vi "USB6343_Control.vi"(11 "monitor buff":refnum<vi>) -> (0 "error out":errorcluster, 3 "msg interface":refnum<user-event>)   [LabVIEW 2013]
uses:
  <vilib>/DAQmx/write.llb/DAQmx Write.vi
  <vilib>/DAQmx/write.llb/DAQmx Write (Digital 1D Bool NChan 1Samp 1Line).vi
  <vilib>/DAQmx/write.llb/DAQmx Write (Analog 1D DBL NChan 1Samp).vi
  <vilib>/DAQmx/read.llb/DAQmx Read.vi
  <vilib>/DAQmx/read.llb/DAQmx Read (Analog 1D DBL NChan 1Samp).vi
  <vilib>/DAQmx/miscellaneous.llb/DAQmx Fill In Error Info.vi
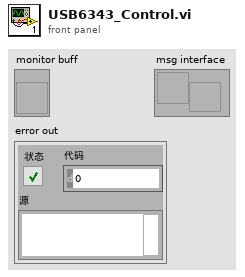
[diagram p1: front panel]
types:
  T1 = cluster{"cmd":string, "value":dbl, "result ":refnum<vi>, "channel":i32, "on/off":bool}
  T2 = cluster{"AI Task":refnum<k21>, "AO Task":refnum<k21>, "DO Task":refnum<k21>}
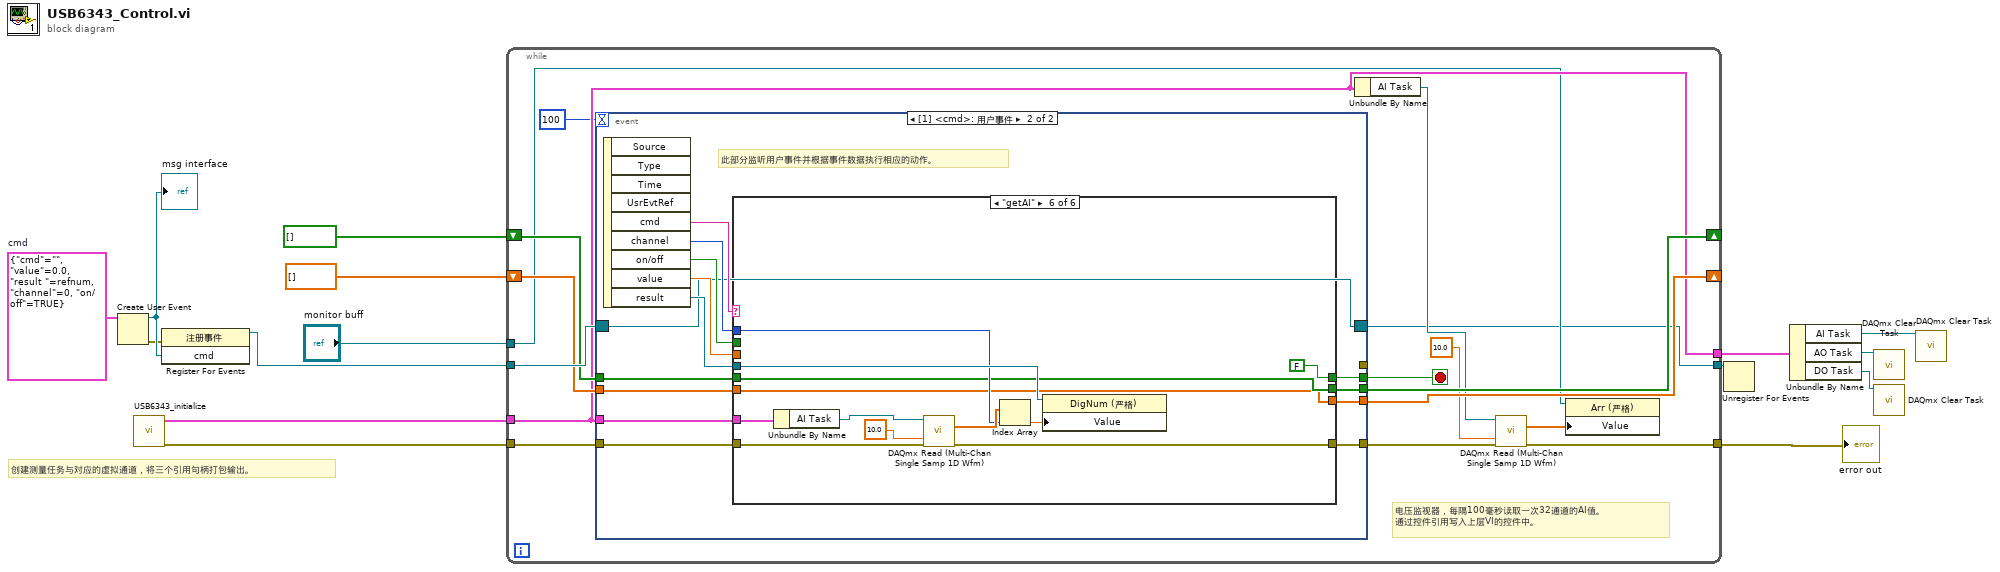
[diagram p0: block diagram]
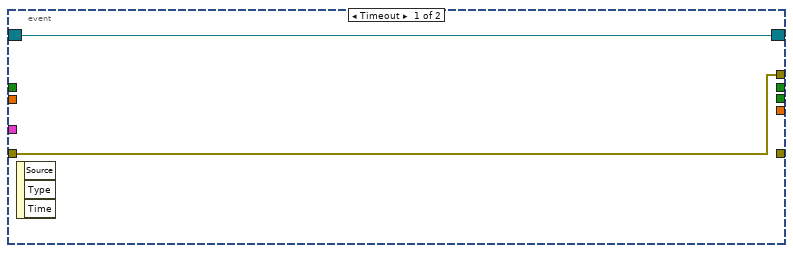
[diagram p2: hidden frame]
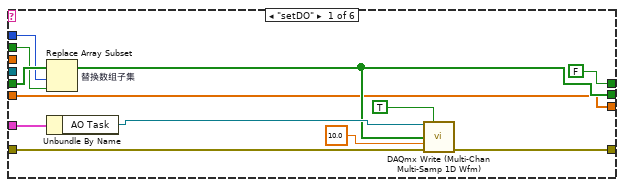
[diagram p3: hidden frame]
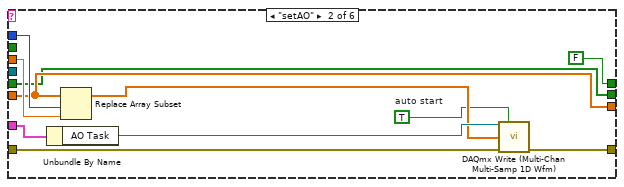
[diagram p4: hidden frame]
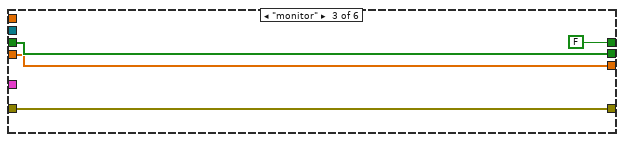
[diagram p5: hidden frame]
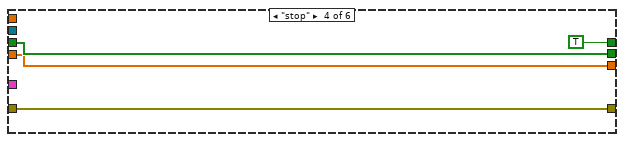
[diagram p6: hidden frame]
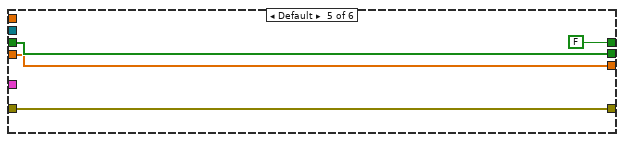
[diagram p7: hidden frame]
diagram:
  w10 = T1 {"cmd"="", "value"=0.0, "result "=refnum, "channel"=0, "on/off"=TRUE}  # cmd
  # "创建测量任务与对应的虚拟通道，将三个引用句柄打包输出。"
  n1 = Create User Event(user event datatype=w10) -> (user event=w15:refnum<user-event>, error out=w14:errorcluster)  [unwired: 1 in]
  "msg interface" <- w15
  n2 = call "USB6343_initialize.vi"() -> ("error out"=w12:errorcluster, "Tasks"=w13:T2)  [unwired: 10 in]
  n3 = register-events(error in=w14, w15) -> (reference out=w11:refnum<event-registration>)  [unwired: 1 in, 1 out]
  n4 = while {
    tunnel: w13 -> [w24]
    tunnel: w12 -> [w31]
    tunnel: w11 -> [w30]
    shift-right: [w28] -> _
    shift-left: bool[] [] ("data") -> [w29]
    tunnel: [w24] -> w8
    shift-right: [w25] -> _
    shift-left: dbl[] [] ("data") -> [w26]
    tunnel: "monitor buff" -> [w20]
    tunnel: [w18] -> w3
    tunnel: [w16] -> w1
    stop <- w27 stop-if-true
    # "电压监视器，每隔100毫秒读取一次32通道的AI值。\n通过控件引用写入上层VI的控件中。"
    n5 = event shown="[1] <cmd>: 用户事件" {
      selector: w30 -> [w32 w34]
      dyn-events: [w32 w34] -> w16
      timeout: 100 -> [_ _]
      tunnel: w24 -> [_ w46]
      tunnel: [w33 _] -> _
      tunnel: w31 -> [w33 w45]
      tunnel: w29 -> [_ w44]
      tunnel: [_ w42] -> w28
      tunnel: [_ w40] -> w27
      tunnel: w26 -> [_ w39]
      tunnel: [_ w37] -> w25
      tunnel: [_ w35] -> w21
      event Timeout {
        n6 = event-data() -> ()  [unwired: 1 in, 3 out]
      }
      event User Event {
        # "此部分监听用户事件并根据事件数据执行相应的动作。"
        n7 = event-data() -> ("cmd"=w41:string, "channel"=w47:i32, "on/off"=w43:bool, "value"=w38:dbl, "result"=w36:refnum<vi>)  [unwired: 1 in, 4 out]
        n8 = case shown="\"getAI\"" w41 {
          tunnel: w47 -> [w53 w68 _ _ _ w88]
          tunnel: w46 -> [w59 w70 _ _ _ w94]
          tunnel: w45 -> [w56 w60 w71 w75 w79 w90]
          tunnel: w44 -> [w54 w65 w74 w78 w82 w86]
          tunnel: w43 -> [w52 _ _ _ _ _]
          tunnel: [w51 w65 w74 w78 w82 w86] -> w42
          tunnel: [FALSE FALSE FALSE TRUE FALSE FALSE] -> w40
          tunnel: w39 -> [w49 w66 w73 w76 w80 w85]
          tunnel: w38 -> [_ w67 _ _ _ _]
          tunnel: [w49 w66 w73 w76 w80 w85] -> w37
          tunnel: w36 -> [_ _ _ _ _ w92]
          tunnel: [w48 w61 w71 w75 w79 w83] -> w35
          frame "setDO" {
            n9 = Replace Array Subset "替换数组子集"(array=w54, new element=w52, index=w53) -> (w51:bool[])
            n10 = Unbundle By Name(w59) -> ("AO Task"=w58:refnum<k21>)
            n11 = call-poly "DAQmx Write (Multi-Chan Multi-Samp 1D Wfm).vi"("task/channels in"=w58, "auto start"=TRUE, "data"=w51, "timeout"=10.0, "error in"=w56) -> ("error out"=w48:errorcluster)  [unwired: 8 in, 2 out]
          }
          frame "setAO" {
            w63 = TRUE  # auto start
            n12 = Unbundle By Name(w70) -> ("AO Task"=w69:refnum<k21>)
            n13 = Replace Array Subset(array=w66, new element=w67, index=w68) -> (w64:dbl[])
            n14 = call-poly "DAQmx Write (Multi-Chan Multi-Samp 1D Wfm).vi"("task/channels in"=w69, "auto start"=w63, "data"=w64, "error in"=w60) -> ("error out"=w61:errorcluster)  [unwired: 9 in, 2 out]
          }
          frame "monitor" {
          }
          frame "stop" {
          }
          frame Default {
          }
          frame "getAI" {
            n15 = Unbundle By Name(w94) -> ("AI Task"=w93:refnum<k21>)
            n16 = call-poly "DAQmx Read (Multi-Chan Single Samp 1D Wfm).vi"("task/channels in"=w93, "timeout"=10.0, "error in"=w90) -> ("data"=w89:dbl[], "error out"=w83:errorcluster)  [unwired: 10 in, 1 out]
            n17 = Index Array(array=w89, index=w88) -> (element=w87:dbl)
            n18 = property class="DigNum (严格)"(reference=w92, "Value"=w87) -> ()  [unwired: 1 in, 2 out]
          }
        }
      }
    }
    n19 = Unbundle By Name(w24) -> ("AI Task"=w23:refnum<k21>)
    n20 = call-poly "DAQmx Read (Multi-Chan Single Samp 1D Wfm).vi"("task/channels in"=w23, "timeout"=10.0, "error in"=w21) -> ("data"=w19:dbl[], "error out"=w18:errorcluster)  [unwired: 10 in, 1 out]
    n21 = property class="Arr (严格)"(reference=w20, "Value"=w19) -> ()  [unwired: 1 in, 2 out]
  }
  "error out" <- w3
  n22 = Unregister For Events(event registration refnum=w1) -> ()  [unwired: 1 in, 1 out]
  n23 = Unbundle By Name(w8) -> ("AI Task"=w7:refnum<k21>, "AO Task"=w6:refnum<k21>, "DO Task"=w5:refnum<k21>)
  n24 = call <vilib>:"DAQmx Clear Task.vi"("task in"=w6) -> ()  [unwired: 14 in, 1 out]
  n25 = call <vilib>:"DAQmx Clear Task.vi"("task in"=w5) -> ()  [unwired: 14 in, 1 out]
  n26 = call <vilib>:"DAQmx Clear Task.vi"("task in"=w7) -> ()  [unwired: 14 in, 1 out]
